vi "未命名 2.vi"() -> ()   [LabVIEW 2018]
panel:
  out "波形图":dynamicdata(graph)
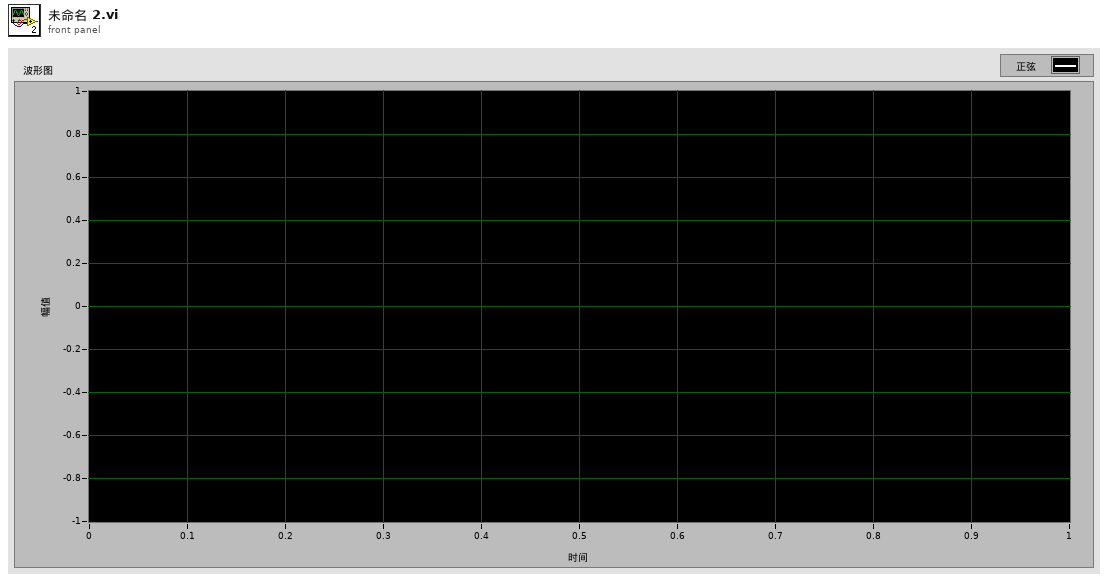
[diagram p1: front panel]
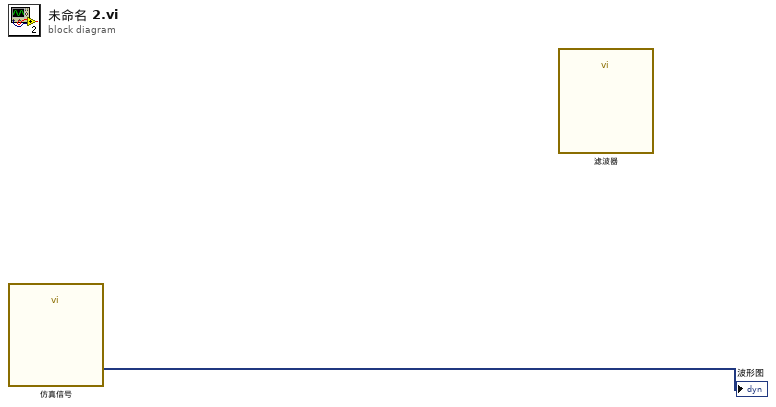
[diagram p0: block diagram]
diagram:
  n1 = call "仿真信号"() -> ("正弦"=→"波形图":dynamicdata)  [unwired: 14 in, 1 out]
  n2 = call "滤波器"() -> ()  [unwired: 10 in, 2 out]
